vi "Get Directory Receusively.vi"(10 "path":path, 11 "Map":map{path, cluster{"size":i64, "file count":i32}}(c390)) -> (1 "size":i64, 2 "file count":i32, 3 "map out":map{path, cluster{"size":i64, "file count":i32}}(c390))   [LabVIEW 2023]
panel:
  out "error out":errorcluster
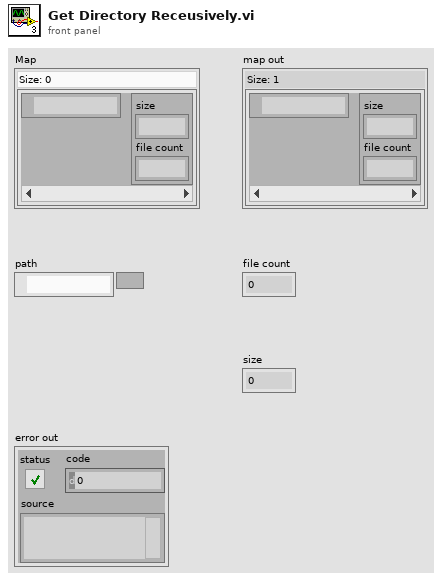
[diagram p1: front panel]
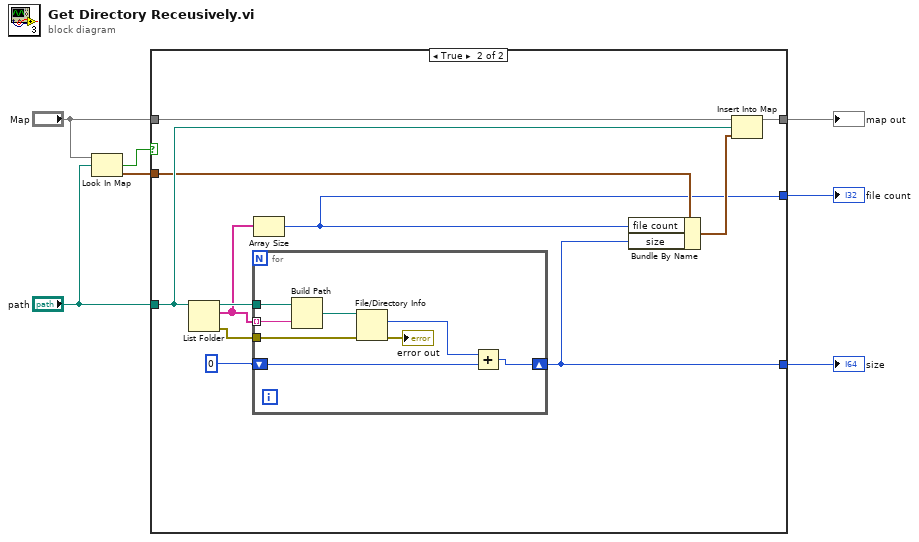
[diagram p0: block diagram]
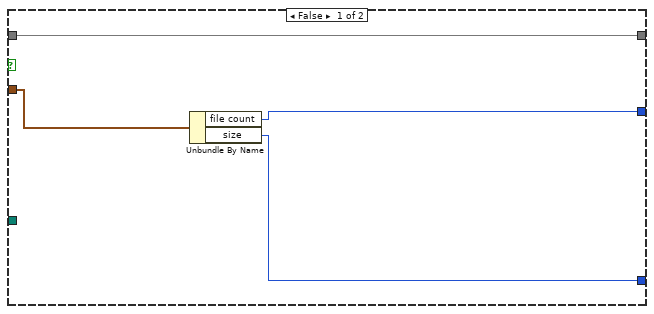
[diagram p2: hidden frame]
diagram:
  n1 = Look In Map(map="Map", key="path") -> (key not found?=w3:bool, value=w5:cluster{"size":i64, "file count":i32})  [unwired: 1 in]
  n2 = case shown="True" w3 {
    tunnel: "Map" -> [w11 w21]
    tunnel: "path" -> [_ w20]
    tunnel: w5 -> [w10 w18]
    tunnel: [w11 w16] -> w4
    tunnel: [w8 w14] -> w2
    tunnel: [w9 w13] -> w1
    frame False {
      n3 = Unbundle By Name(w10) -> ("file count"=w9:i32, "size"=w8:i64)
    }
    frame True {
      n4 = List Folder(path=w20) -> (path out=w22:path, filenames=w19:string[], error out=w12:errorcluster)  [unwired: 2 in, 2 out]
      n5 = for {
        tunnel: w22 -> [w24]
        tunnel: w19 -> [w28] mode=indexing
        shift-right: [w25] -> w14
        shift-left: i64 0 -> [w26]
        tunnel: w12 -> [w23]
        n6 = Build Path(base path=w24, name or relative path=w28) -> (appended path=w27:path)
        n7 = File/Directory Info(path=w27, error in=w23) -> (size=w30:i64, error out=→"error out":errorcluster)  [unwired: 5 out]
        n8 = Add(x=w30, y=w26) -> (x+y=w25:i64)
      }
      n9 = Array Size(array=w19) -> (size(s)=w13:i32)
      n10 = Bundle By Name(cluster=w18, "file count"=w13, "size"=w14) -> (w17:cluster{"size":i64, "file count":i32})
      n11 = Insert Into Map(map in=w21, key=w20, value=w17) -> (map out=w16:map{path, cluster{"size":i64, "file count":i32}})  [unwired: 2 out]
    }
  }
  "map out" <- w4
  "size" <- w2
  "file count" <- w1
